vi "Do_ADAM_channel.vi"(4 "Scan Period":dbl format="%.2f", 5 "Previous Scan Value":dbl format="%.2f", 6 "Present scan array":dbl[](array[numeric]) format="%.2f", 7 "Value to Output":dbl format="%.2f", 8 "Ch Description":T1={"Ch Name"="", "Type"=enum."Test", "Function"=enum."Analogue Input", "Ch State"=enum."On", "Calibration type"=enum."Raw", "A"=0.0, "B"=0.0, "C"=0.0, "D"=0.0, "Comments"="", "Address"={"Main"=0, "Ch."=0, "Sub"=0, "Port Name"=""}, "String"="", "Duty"=0} {"Duty" format="%.0b"; "D" format="%#_5g"; "C" format="%#_5g"; "B" format="%#_5g"; "A" format="%#_5g"}, 9 "Ch names":string[](array[string])) -> (0 "Scan comment":string, 1 "Output":dbl format="%.3f")   [LabVIEW 2010]
uses:
  ADAM Client/Sub VIs/ADAM Controls/Ch_description_ADAM.ctl
  ADAM Client/Sub VIs/ADAM Controls/Module_type_ADAM.ctl
  ADAM Client/Sub VIs/ADAM Controls/Function_ADAM.ctl
  ADAM Client/Sub VIs/ADAM Controls/Channel_State.ctl
  ADAM Client/Sub VIs/ADAM Controls/Calib_type_ADAM.ctl
  ADAM Client/Sub VIs/ADAM Controls/Address.ctl
  ADAM Client/Sub VIs/ADAM Controls/Remember_value_mode.ctl
  ADAM Client/Sub VIs/ADAM Controls/Search_mode.ctl
  Anemometry/Anemometry Sub Vis/Controls/In_Range.ctl
  Anemometry/Anemometry Sub Vis/Globals/Gas_management_global.vi
  ADAM_Global.vi
  Anemometry/Anemometry Sub Vis/Globals/Constants_global.vi
panel:
  in  "Case Constant\n(See Context Help) 2":bool=TRUE
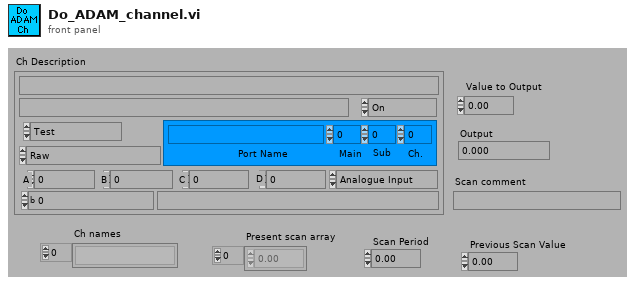
[diagram p1: front panel]
types:
  T1 = typedef "Ch_description_ADAM.ctl" = cluster{"Ch Name":string, "Type":T2, "Function":T3, "Ch State":T4, "Calibration type":T5, "A":dbl, "B":dbl, "C":dbl, "D":dbl, "Comments":string, "Address":T6, "String":string, "Duty":u16}
  T2 = typedef "Module_type_ADAM.ctl" = enum16{"4011", "4012", "4013", "4014", "4016", "4017", "4018", "4021", "4050", "4052", "4053", "4060", "4080", "5000", "5017", "5018", "5024", "5051", "5056", "5060", "6060", "Tracker", "WEST", "GILL", "JEM", "VICI", "Vaisala", "DRUCK", "Run VI Named:", "IR2100", "PPT", "Comparator", "VIRTUAL", "Hold Value", "Read A", "Read Ch", "Coded", "Client Info", "Web Client", "X10", "Test"}
  T3 = typedef "Function_ADAM.ctl" = enum16{"Analogue Input", "Digital Input", "Event counter", "Event rate", "Analogue Output", "Digital Output", "Relay Output"}
  T4 = typedef "Channel_State.ctl" = enum16{"On", "Off", "Always On", "Always Off"}
  T5 = typedef "Calib_type_ADAM.ctl" = enum16{"Raw", "Bx + A", "Cx^2 + Bx + A", "Dx^3 + Cx^2 + Bx + A", "In Band", "Hi-Tec Q", "Hi-Tec M_dot", "Text"}
  T6 = typedef "Address.ctl" = cluster{"Main":i32, "Ch.":i32, "Sub":i32, "Port Name":string}
  T7 = typedef "Remember_value_mode.ctl" = enum16{"Read only", "Read and Write"}
  T8 = typedef "Search_mode.ctl" = enum16{"Between times", "All Times"}
  T9 = typedef "In_Range.ctl" = enum16{"%", "±", "% & ±"}
  T10 = typedef "Valco_valve_ph.ctl" = u16
  T11 = cluster{"Centre Times":dbl[], "Output array":dbl[]}
  T12 = cluster{"Centre Times":dbl[], "Output array":dbl[]}[]
  T13 = typedef "LVDateTimeRec.ctl" = cluster{"fractional second":dbl, "second":i32, "minute":i32, "hour":i32, "day of month":i32, "month":i32, "year":i32, "day of week":i32, "day of year":i32, "DST":i32}
  T14 = typedef "Client_State_Cluster.ctl" = cluster{"Client Name":string, "Traverse level State":T15, "People to Email":string[], "Next Contact Time":dbl}
  T15 = typedef "Traverse_Level_State.ctl" = enum16{"Running", "Complete"}
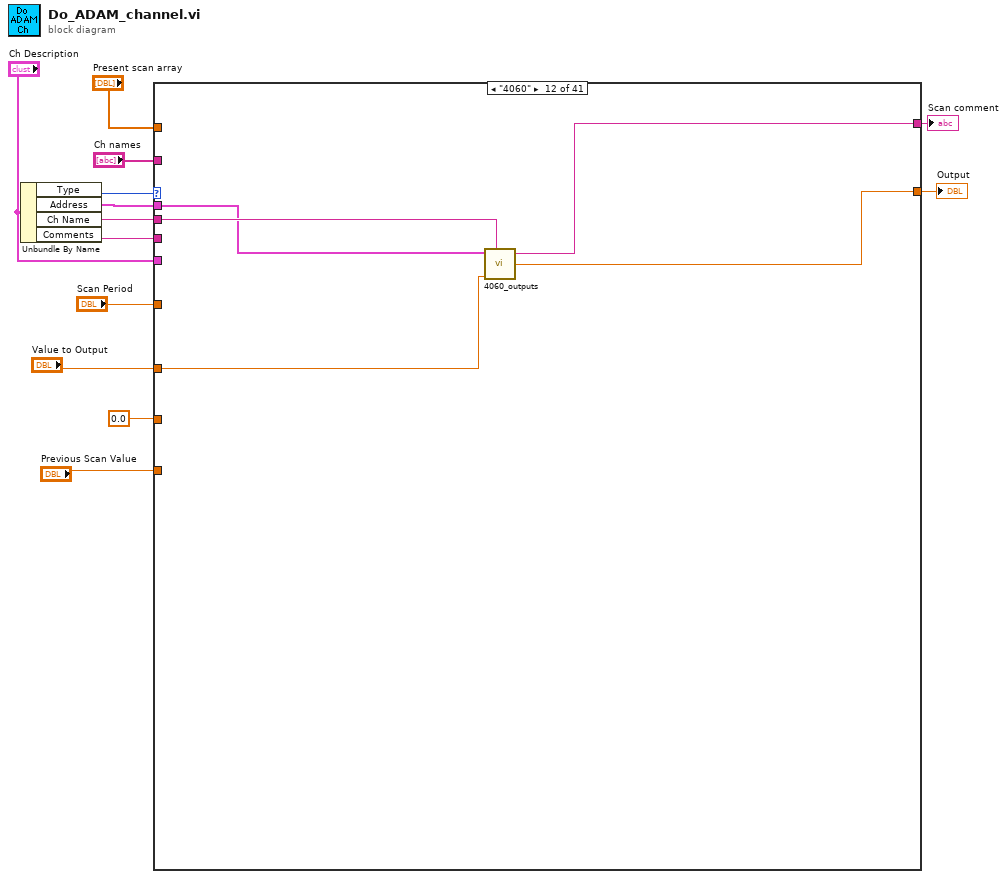
[diagram p0: block diagram]
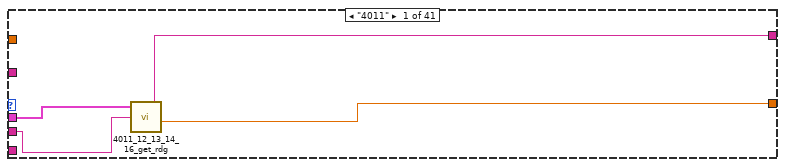
[diagram p2: hidden frame]
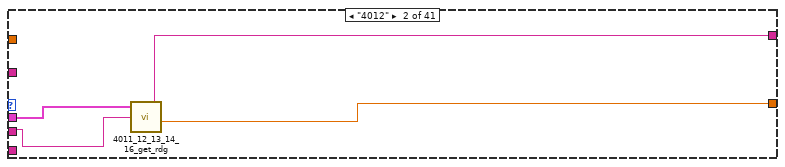
[diagram p3: hidden frame]
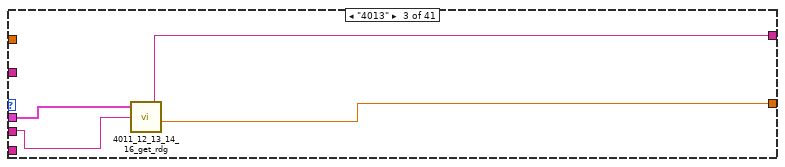
[diagram p4: hidden frame]
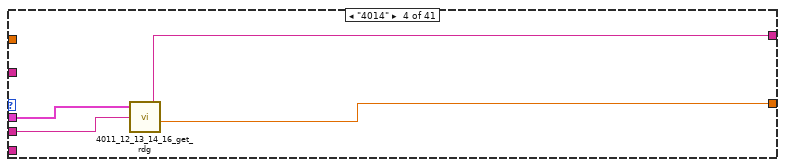
[diagram p5: hidden frame]
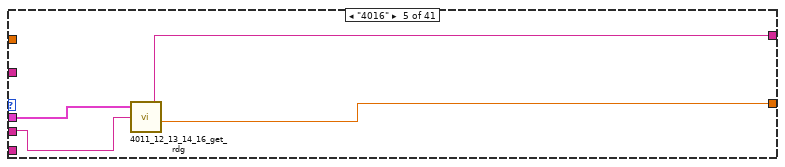
[diagram p6: hidden frame]
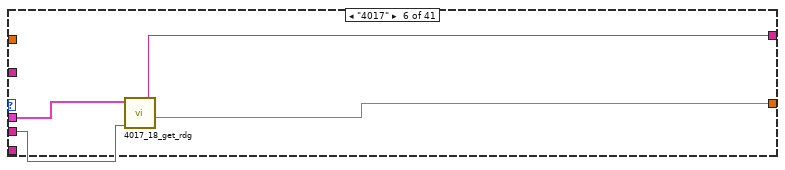
[diagram p7: hidden frame]
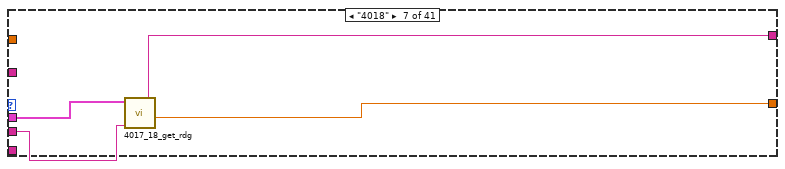
[diagram p8: hidden frame]
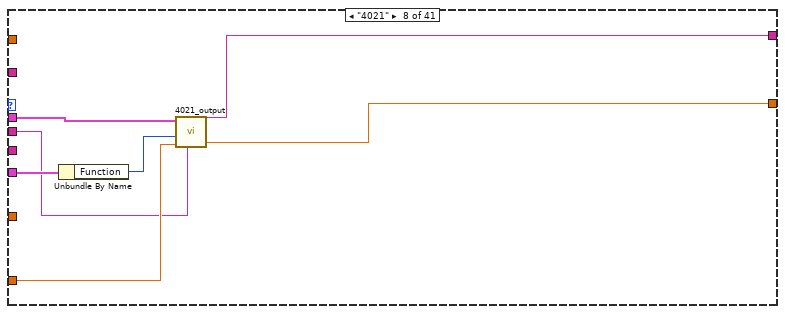
[diagram p9: hidden frame]
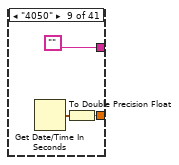
[diagram p10: hidden frame]
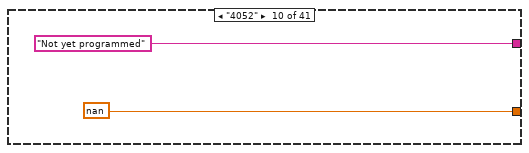
[diagram p11: hidden frame]
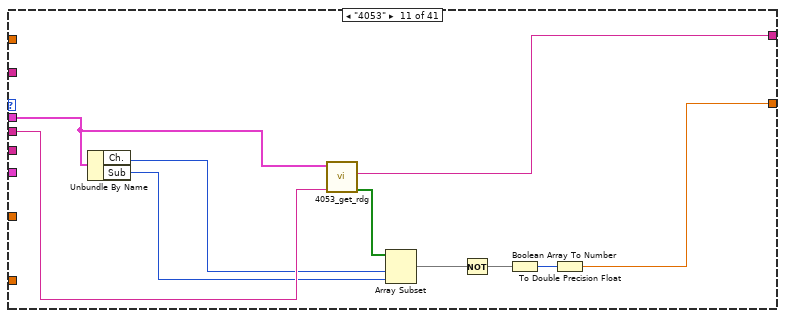
[diagram p12: hidden frame]
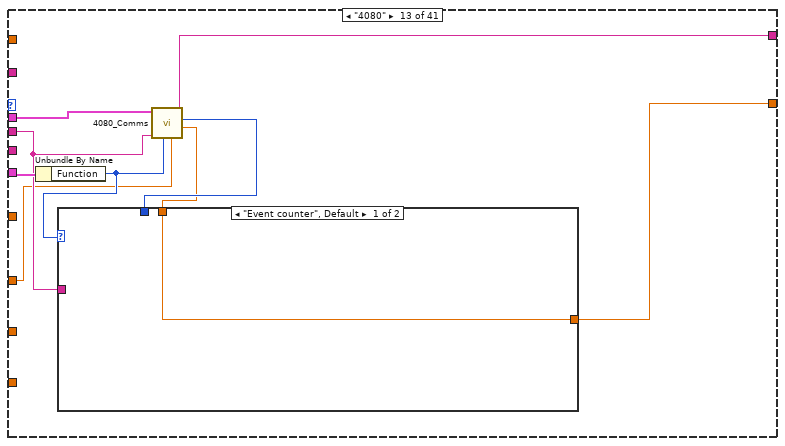
[diagram p13: hidden frame]
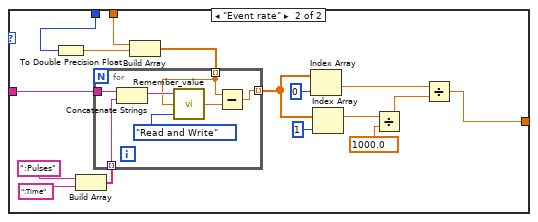
[diagram p14: hidden frame]
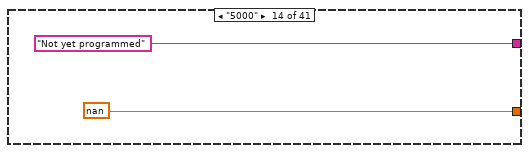
[diagram p15: hidden frame]
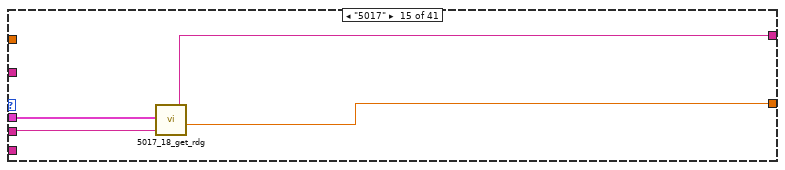
[diagram p16: hidden frame]
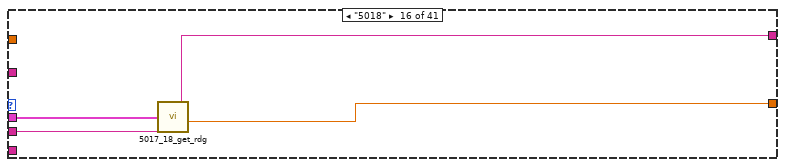
[diagram p17: hidden frame]
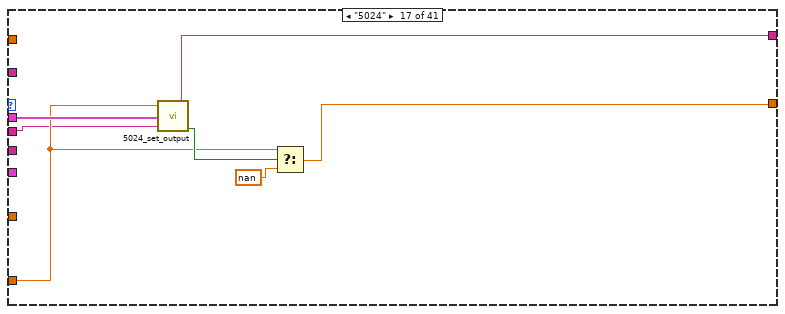
[diagram p18: hidden frame]
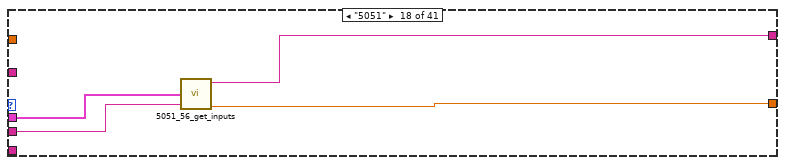
[diagram p19: hidden frame]
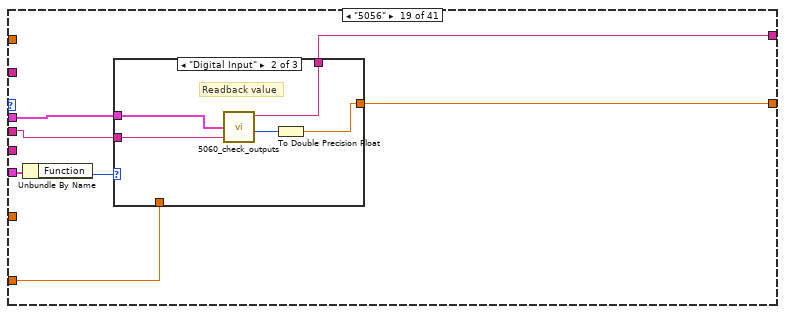
[diagram p20: hidden frame]
diagram:
  n1 = Unbundle By Name("Ch Description") -> ("Type"=w11:T2, "Address"=w10:T6, "Ch Name"=w2:string, "Comments"=w7:string)
  n2 = case shown="\"4060\"" w11 {
    tunnel: [w16 w20 w24 w28 w32 w36 w40 w47 w50 nan w57 w66 w75 nan w105 w109 w114 w120 w128 w149 w171 w190 nan w258 w271 w296 w335 nan w347 w378 w383 w384 w496 w920 w922 w926 w931 w943 w977 w1003 w1017] -> w8
    tunnel: [w17 w21 w25 w29 w33 w37 w41 w48 "" "Not yet programmed" w62 w67 w77 "Not yet programmed" w106 w110 w117 w121 w127 w150 w172 w192 "Not yet programmed" w257 w270 w288 w336 "Not yet programmed" w346 w379 w382 w405 w495 "" "" w927 "" "" w966 "" w1016] -> w5
    tunnel: w10 -> [w14 w18 w22 w26 w30 w34 w38 w42 _ _ w54 w65 w69 _ w107 w111 w118 w122 w126 w151 w173 w194 _ w255 w275 w293 w341 _ _ w377 w380 _ w487 _ _ _ _ _ _ w1012 w1015]
    tunnel: "Ch Description" -> [_ _ _ _ _ _ _ w46 _ _ _ _ w76 _ _ _ _ _ w125 w148 w170 w193 _ _ _ _ _ _ w352 _ _ w410 w489 _ w923 w928 _ _ _ _ _]
    tunnel: w2 -> [w15 w19 w23 w27 w31 w35 w39 w43 _ _ w63 w68 w72 _ w104 w108 w112 w119 w123 w145 w167 w191 _ w256 w273 w289 w340 _ _ _ w381 _ w492 _ _ _ _ w939 w973 _ w1014]
    tunnel: "Ch names" -> [_ _ _ _ _ _ _ _ _ _ _ _ _ _ _ _ _ _ _ _ _ _ _ _ _ _ _ _ w353 _ _ w409 w494 _ _ w929 _ _ _ _ _]
    tunnel: "Present scan array" -> [_ _ _ _ _ _ _ _ _ _ _ _ _ _ _ _ _ _ _ _ _ _ _ _ _ _ _ _ w350 _ _ w407 w493 _ _ w930 _ _ _ _ _]
    tunnel: w7 -> [_ _ _ _ _ _ _ _ _ _ _ _ _ _ _ _ _ _ _ _ _ _ _ _ _ _ _ _ w345 _ _ w411 _ _ _ _ _ _ _ _ _]
    tunnel: "Value to Output" -> [_ _ _ _ _ _ _ w44 _ _ _ w64 w70 _ _ _ w113 _ w124 w146 w168 w189 _ _ w259 w297 _ _ w351 _ _ _ _ _ _ _ _ _ _ w1007 _]
    tunnel: "Scan Period" -> [_ _ _ _ _ _ _ _ _ _ _ _ _ _ _ _ _ _ _ _ _ _ _ _ _ _ _ _ w348 _ _ _ w491 _ _ _ _ _ _ _ _]
    tunnel: "Previous Scan Value" -> [_ _ _ _ _ _ _ _ _ _ _ _ _ _ _ _ _ _ _ _ _ _ _ _ _ _ _ _ w349 _ _ w385 w490 w920 _ _ w931 _ _ _ _]
    tunnel: 0.0 -> [_ _ _ _ _ _ _ _ _ _ _ _ _ _ _ _ _ _ _ _ _ _ _ _ _ _ _ _ _ _ _ _ w488 _ _ _ _ _ _ _ _]
    frame "4011" {
      n3 = call "4011_12_13_14_16_get_rdg.vi"("Address"=w14, "Channel Name"=w15) -> ("Comment"=w17:string, "Reading"=w16:dbl)  [unwired: 1 in, 2 out]
    }
    frame "4012" {
      n4 = call "4011_12_13_14_16_get_rdg.vi"("Address"=w18, "Channel Name"=w19) -> ("Comment"=w21:string, "Reading"=w20:dbl)  [unwired: 1 in, 2 out]
    }
    frame "4013" {
      n5 = call "4011_12_13_14_16_get_rdg.vi"("Address"=w22, "Channel Name"=w23) -> ("Comment"=w25:string, "Reading"=w24:dbl)  [unwired: 1 in, 2 out]
    }
    frame "4014" {
      n6 = call "4011_12_13_14_16_get_rdg.vi"("Address"=w26, "Channel Name"=w27) -> ("Comment"=w29:string, "Reading"=w28:dbl)  [unwired: 1 in, 2 out]
    }
    frame "4016" {
      n7 = call "4011_12_13_14_16_get_rdg.vi"("Address"=w30, "Channel Name"=w31) -> ("Comment"=w33:string, "Reading"=w32:dbl)  [unwired: 1 in, 2 out]
    }
    frame "4017" {
      n8 = call "4017_18_get_rdg.vi"("Channel Name"=w35, "Address"=w34) -> ("Reading"=w36:dbl, "Comment"=w37:string)  [unwired: 2 in, 2 out]
    }
    frame "4018" {
      n9 = call "4017_18_get_rdg.vi"("Channel Name"=w39, "Address"=w38) -> ("Reading"=w40:dbl, "Comment"=w41:string)  [unwired: 2 in, 2 out]
    }
    frame "4021" {
      n10 = Unbundle By Name(w46) -> ("Function"=w45:T3)
      n11 = call "4021_output.vi"("Address"=w42, "Function"=w45, "Set to:"=w44, "Channel Name"=w43) -> ("Comment"=w48:string, "Reading"=w47:dbl)  [unwired: 1 in, 1 out]
    }
    frame "4050" {
      n12 = Get Date/Time In Seconds() -> (seconds since 1Jan1904=w49:timestamp)
      n13 = To Double Precision Float(number=w49) -> (double precision float=w50:dbl)
    }
    frame "4052" {
    }
    frame "4053" {
      n14 = Unbundle By Name(w54) -> ("Ch."=w55:i32, "Sub"=w61:i32)
      n15 = call "4053_get_rdg.vi"("Channel Name"=w63, "Address"=w54) -> ("Boolean array"=w60:bool[], "Comment"=w62:string)  [unwired: 2 in, 2 out]
      n16 = Array Subset(array=w60, index=w55, length=w61) -> (w59:bool[])
      n17 = Not(x=w59) -> (.not. x?=w56:bool[])
      n18 = Boolean Array To Number(Boolean array=w56) -> (number=w58:u32)
      n19 = To Double Precision Float(number=w58) -> (double precision float=w57:dbl)
    }
    frame "4060" {
      n20 = call "4060_outputs.vi"("Address"=w65, "Value to Output"=w64, "Channel Name"=w68) -> ("Comment"=w67:string, "Reading"=w66:dbl)  [unwired: 2 in, 1 out]
    }
    frame "4080" {
      n21 = Unbundle By Name(w76) -> ("Function"=w71:T3)
      n22 = call "4080_Comms.vi"("Value to display"=w70, "Function"=w71, "Channel Name"=w72, "Address"=w69) -> ("Reading"=w73:dbl, "millisecond timer value"=w74:u32, "Comment"=w77:string)  [unwired: 2 in, 1 out]
      n23 = case shown="\"Event counter\", Default" w71 {
        tunnel: w72 -> [_ w94]
        tunnel: w74 -> [_ w87]
        tunnel: [w78 w79] -> w75
        tunnel: w73 -> [w78 w88]
        frame "Event counter", Default {
        }
        frame "Event rate" {
          n24 = To Double Precision Float(number=w87) -> (double precision float=w86:dbl)
          n25 = Build Array(":Pulses", ":Time") -> (w89:string[])
          n26 = Build Array(w88, w86) -> (w85:dbl[])
          n27 = for {
            tunnel: w94 -> [w98]
            tunnel: [w99] -> w82 mode=indexing
            tunnel: w89 -> [w96] mode=indexing
            tunnel: w85 -> [w95] mode=indexing
            n28 = Concatenate Strings(w98, w96) -> (w97:string)
            n29 = call "Remember_value.vi"("Mode"=Remember_value_mode."Read and Write", "Input Value"=w95, "Ch name"=w97) -> ("Output Value"=w100:dbl)
            n30 = Subtract(x=w95, y=w100) -> (x-y=w99:dbl)
          }
          n31 = Index Array(array=w82, index=0) -> (element=w80:dbl)
          n32 = Index Array(array=w82, index=1) -> (element=w81:dbl)
          n33 = Divide(x=w81, y=1000.0) -> (x/y=w92:dbl)
          n34 = Divide(x=w80, y=w92) -> (x/y=w79:dbl)
        }
      }
    }
    frame "5000" {
    }
    frame "5017" {
      n35 = call "5017_18_get_rdg.vi"("Address (all reqd.)"=w107, "Channel Name"=w104) -> ("Comment"=w106:string, "Reading"=w105:dbl)  [unwired: 3 out]
    }
    frame "5018" {
      n36 = call "5017_18_get_rdg.vi"("Address (all reqd.)"=w111, "Channel Name"=w108) -> ("Comment"=w110:string, "Reading"=w109:dbl)  [unwired: 3 out]
    }
    frame "5024" {
      n37 = call "5024_set_output.vi"("Set to:"=w113, "Address (all reqd.)"=w118, "Channel Name"=w112) -> ("Comment"=w117:string, "Good Reply"=w115:bool)  [unwired: 2 out]
      n38 = Select(t=w113, s=w115, f=nan) -> (s? t:f=w114:dbl)
    }
    frame "5051" {
      n39 = call "5051_56_get_inputs.vi"("Address (Main, Sub reqd.)"=w122, "Channel Name"=w119) -> ("Comment"=w121:string, "Single output"=w120:dbl)  [unwired: 3 out]
    }
    frame "5056" {
      n40 = Unbundle By Name(w125) -> ("Function"=w129:T3)
      n41 = case shown="\"Digital Input\"" w129 {
        tunnel: w126 -> [_ w135 w144]
        tunnel: ["This function is not available" w136 w142] -> w127
        tunnel: [nan ("A") w133 w139] -> w128
        tunnel: w124 -> [_ _ w138]
        tunnel: w123 -> [_ w132 w137]
        frame "Analogue Input", Default {
        }
        frame "Digital Input" {
          # "Readback value"
          n42 = call "5060_check_outputs.vi"("Address (Main, Sub reqd.)"=w135, "Channel Name"=w132) -> ("Comment"=w136:string, "Single Channel"=w134:i16)  [unwired: 3 out]
          n43 = To Double Precision Float(number=w134) -> (double precision float=w133:dbl)
        }
        frame "Relay Output" {
          # "Sets single o/p channel"
          n44 = Greater Than 0?(x=w138) -> (x > 0?=w143:bool)
          n45 = call "5056_60_set_single_output.vi"("Channel Name"=w137, "Address (all reqd.)"=w144, "Set state:"=w143) -> ("Comment"=w142:string, "Good Reply"=w141:bool)  [unwired: 2 out]
          n46 = Select(t=w138, s=w141, f=nan) -> (s? t:f=w139:dbl)
        }
      }
    }
    frame "5060" {
      n47 = Unbundle By Name(w148) -> ("Function"=w147:T3)
      n48 = case shown="\"Relay Output\"" w147 {
        tunnel: w151 -> [_ w157 w166]
        tunnel: ["This function is not available" w158 w164] -> w150
        tunnel: [nan ("A") w155 w161] -> w149
        tunnel: w146 -> [_ _ w160]
        tunnel: w145 -> [_ w154 w159]
        frame "Analogue Input", Default {
        }
        frame "Digital Input" {
          # "Readback value"
          n49 = call "5060_check_outputs.vi"("Address (Main, Sub reqd.)"=w157, "Channel Name"=w154) -> ("Comment"=w158:string, "Single Channel"=w156:i16)  [unwired: 3 out]
          n50 = To Double Precision Float(number=w156) -> (double precision float=w155:dbl)
        }
        frame "Relay Output" {
          # "Sets single o/p channel"
          n51 = Greater Than 0?(x=w160) -> (x > 0?=w165:bool)
          n52 = call "5056_60_set_single_output.vi"("Channel Name"=w159, "Address (all reqd.)"=w166, "Set state:"=w165) -> ("Comment"=w164:string, "Good Reply"=w163:bool)  [unwired: 2 out]
          n53 = Select(t=w160, s=w163, f=nan) -> (s? t:f=w161:dbl)
        }
      }
    }
    frame "6060" {
      n54 = Unbundle By Name(w170) -> ("Function"=w169:T3)
      n55 = case shown="\"Digital Input\"" w169 {
        tunnel: w173 -> [_ w179 w188]
        tunnel: ["This function is not available" w180 w186] -> w172
        tunnel: [nan ("A") w177 w183] -> w171
        tunnel: w168 -> [_ _ w182]
        tunnel: w167 -> [_ w176 w181]
        frame "Analogue Input", Default {
        }
        frame "Digital Input" {
          n56 = call "6060_read_all_I-O.vi"("Address (Main, Sub reqd.)"=w179, "Channel Name"=w176) -> ("Comment"=w180:string, "Single Input Channel"=w178:i16)  [unwired: 3 out]
          n57 = To Double Precision Float(number=w178) -> (double precision float=w177:dbl)
        }
        frame "Relay Output" {
          # "Sets single o/p channel"
          n58 = Greater Than 0?(x=w182) -> (x > 0?=w187:bool)
          n59 = call "6060_set_single_output.vi"("Channel Name"=w181, "Address (Main, Ch requd.)"=w188, "Set state:"=w187) -> ("Comment"=w186:string, "Good Reply"=w185:bool)  [unwired: 2 out]
          n60 = Select(t=w182, s=w185, f=nan) -> (s? t:f=w183:dbl)
        }
      }
    }
    frame "Tracker" {
      n61 = while {
        tunnel: w194 -> [w218]
        tunnel: w193 -> [w217]
        tunnel: [w211] -> w192
        tunnel: w191 -> [w210]
        tunnel: [w204] -> w190
        tunnel: w189 -> [w203]
        i -> [w200]
        stop <- w197 continue-if-true
        n62 = Unbundle By Name(w217) -> ("Function"=w216:T3)
        n63 = Unbundle By Name(w218) -> ("Port Name"=w215:string, "Ch."=w206:i32, "Main"=w214:i32, "Sub"=w213:i32)
        n64 = case shown="\"Analogue Output\"" w216 {
          tunnel: [enum16{"Set", "Read"}."Set" ("Set") enum16{"Set", "Read"}."Set" ("Set") enum16{"Set", "Read"}."Set" ("Set") enum16{"Set", "Read"}."Set" ("Set") enum16{"Set", "Read"}."Set" ("Set") enum16{"Set", "Read"}."Read" ("Set") enum16{"Set", "Read"}."Read" ("Set")] -> w201
          tunnel: [enum16{"Logic", "Analogue"}."Analogue" ("Analogue") enum16{"Logic", "Analogue"}."Logic" ("Analogue") enum16{"Logic", "Analogue"}."Logic" ("Analogue") enum16{"Logic", "Analogue"}."Logic" ("Analogue") enum16{"Logic", "Analogue"}."Logic" ("Analogue") enum16{"Logic", "Analogue"}."Logic" ("Analogue") enum16{"Logic", "Analogue"}."Analogue" ("Analogue")] -> w212
          frame "Analogue Output" {
          }
          frame "Digital Output" {
          }
          frame "Relay Output" {
          }
          frame "Event rate" {
          }
          frame "Event counter" {
          }
          frame "Digital Input" {
          }
          frame "Analogue Input" {
          }
        }
        n65 = call "TalkTracker.vi"("PORT NAME"=w215, "Set"=w201, "Channel Name"=w210, "Value to set"=w203, "MODULE ADDRESS"=w214, "LOCATION"=w206, "NO. LOCATIONS"=w213, "Analogue"=w212) -> ("Response"=w208:string, "Good Set?"=w195:bool, "Comment out"=w211:string)  [unwired: 1 in, 4 out]
        n66 = Match Pattern(string=w208, regular expression="\r\n") -> (before substring=w207:string)  [unwired: 4 out]
        n67 = case shown="\"Set\"" w201 {
          tunnel: w207 -> [_ w230]
          tunnel: [w222 w229] -> w205
          tunnel: w203 -> [w224 _]
          tunnel: nan ("Reading") -> [w223 w228]
          tunnel: [w221 w226] -> w198
          tunnel: [0 ("y") 1 ("y")] -> w196
          tunnel: w195 -> [w219 _]
          frame "Set" {
            n68 = Not(x=w219) -> (.not. x?=w221:bool)
            n69 = Select(t=w224, s=w219, f=w223) -> (s? t:f=w222:dbl)
          }
          frame "Read" {
            n70 = String Length(string=w230) -> (length=w232:i32)
            n71 = Fract/Exp String To Number(string=w230, default (0 dbl)=w228) -> (offset past number=w233:i32, number=w231:dbl)  [unwired: 2 out]
            n72 = Equal?(x=w232, y=w233) -> (x = y?=w227:bool)
            n73 = Not(x=w227) -> (.not. x?=w226:bool)
            n74 = Select(t=w231, s=w227, f=w228) -> (s? t:f=w229:dbl)
          }
        }
        n75 = case shown="0, Default" w206 {
          tunnel: w205 -> [w234 w237]
          tunnel: [w234 w235] -> w204
          frame 0, Default {
          }
          frame 283 {
            n76 = Equal To 0?(x=w237) -> (x = 0?=w238:bool)
            n77 = Select(t=nan ("Reading"), s=w238, f=w237) -> (s? t:f=w235:dbl)
          }
        }
        n78 = Less?(x=w200, y=w196) -> (x < y?=w199:bool)
        n79 = And(x=w198, y=w199) -> (x .and. y?=w197:bool)
      }
    }
    frame "WEST" {
    }
    frame "GILL" {
      n80 = call "Gill_get_rdg.vi"("Channel Name"=w256, "Address"=w255) -> ("Output"=w258:dbl, "Status note"=w257:string)  [unwired: 2 in, 2 out]
    }
    frame "JEM" {
      n81 = Unbundle By Name(w275) -> ("Main"=w262:i32, "Ch."=w261:i32, "Port Name"=w274:string)
      n82 = case shown="0, Default" w261 {
        tunnel: [i16[] [-3, -2, -1, 0, 14, 29, 43, 57, 71, 86, 100] i16[] [0, 20, 40, 60, 80, 100, 120]] -> w265
        tunnel: [u8[] [10, 50, 80, 100, 120, 140, 160, 180, 200, 220, 240] u8[] [20, 50, 90, 130, 160, 200, 230]] -> w266
        frame 0, Default {
        }
        frame 1 {
        }
      }
      n83 = Add(x=w262, y=w261) -> (x+y=w260:i32)
      n84 = Threshold 1D Array(2:w259, 3:w265) -> (0:w268:dbl)  [unwired: 1 out]
      n85 = Round To Nearest(number=w268) -> (nearest integer value=w269:dbl)
      n86 = To Long Integer(number=w269) -> (32bit integer=w267:i32)
      n87 = Index Array(array=w266, index=w267) -> (element=w264:u8)
      n88 = call "DMX.vi"("Port Name"=w274, "DMX channel no."=w260, "Set value:"=w264, "Channel Name"=w273) -> ("error"=w272:bool)  [unwired: 2 out]
      n89 = Index Array(array=w265, index=w267) -> (element=w263:i16)
      n90 = case shown="False" w272 {
        tunnel: [w276 nan] -> w271
        tunnel: ["" "Comms Error"] -> w270
        tunnel: w263 -> [w278 _]
        frame False {
          n91 = To Double Precision Float(number=w278) -> (double precision float=w276:dbl)
        }
        frame True {
        }
      }
    }
    frame "VICI" {
      n92 = To Long Integer(number=w297) -> (32bit integer=w292:i32)
      n93 = Unbundle By Name(w293) -> ("Port Name"=w295:string, "Ch."=w294:i32)
      n94 = call "Valco_Valve_Position.vi"("Channel Name"=w289, "Valve Number"=w294, "Port Name"=w295, "Requested Posn."=w292) -> ("Error Message"=w287:string, "Achieved Posn."=w290:T10)  [unwired: 2 out]
      n95 = Empty String/Path?(string/path=w287) -> ()  [unwired: 1 out]
      n96 = case shown="True" TRUE {
        tunnel: w293 -> [w304 _]
        tunnel: w292 -> [w303 _]
        tunnel: [w302 w334] -> w291
        tunnel: w290 -> [_ w334]
        tunnel: w289 -> [w301 _]
        tunnel: [w300 w333] -> w288
        tunnel: w287 -> [_ w333]
        tunnel: w287 -> [w299 _]
        tunnel: "X10" ("Port Name") -> [w298 _]
        frame False {
          n97 = stacked-sequence {
            tunnel: w304 -> [_ _ _ _ _ w325]
            tunnel: w303 -> [_ _ _ _ _ w321]
            tunnel: [_ _ _ _ _ w324] -> w302
            tunnel: w301 -> [_ _ _ _ _ w323]
            tunnel: [_ _ _ _ _ w322] -> w300
            tunnel: w299 -> [_ w310 _ _ _ _]
            tunnel: w298 -> [w305 _ _ w313 _ _]
            frame #0 {
              w307 = 3 items=["-----", "A", "B", "C", "D", "E", "F", "G", "H", "I", "J", "K", "L", "M", "N", "O", "P"] ("House Code")
              n98 = call "X10control.vi"("Port Name"=w305, "Power Request (ON)"=FALSE, "House Code"=w307, "Unit No."=5) -> ()  [unwired: 6 out]
            }
            frame #1 {
              n99 = call "Server_Emails.vi"("Message"=w310, "Contact All clients?"=TRUE, "Subject"="Powering Down FID Valve" ("Error Type")) -> ()  [unwired: 2 in, 3 out]
            }
            frame #2 {
              n100 = Wait (ms)(milliseconds to wait=u32 20000) -> ()  [unwired: 1 out]
            }
            frame #3 {
              w315 = 3 items=["-----", "A", "B", "C", "D", "E", "F", "G", "H", "I", "J", "K", "L", "M", "N", "O", "P"] ("House Code")
              n101 = call "X10control.vi"("Port Name"=w313, "Power Request (ON)"=TRUE, "House Code"=w315, "Unit No."=5) -> ()  [unwired: 6 out]
            }
            frame #4 {
              n102 = Wait (ms)(milliseconds to wait=u32 5000) -> ()  [unwired: 1 out]
            }
            frame #5 {
              n103 = Build Array(1 ("element"), 2 ("element"), w321) -> (w318:i32[])
              n104 = for {
                tunnel: w325 -> [w330]
                tunnel: [w329] -> w324
                tunnel: w323 -> [w328]
                tunnel: [w327] -> w322
                tunnel: w318 -> [w326] mode=indexing
                n105 = Unbundle By Name(w330) -> ("Port Name"=w331:string, "Ch."=w332:i32)
                n106 = call "Valco_Valve_Position.vi"("Channel Name"=w328, "Valve Number"=w332, "Port Name"=w331, "Requested Posn."=w326) -> ("Error Message"=w327:string, "Achieved Posn."=w329:T10)  [unwired: 2 out]
              }
            }
          }
        }
        frame True {
        }
      }
      n107 = To Double Precision Float(number=w291) -> (double precision float=w296:dbl)
    }
    frame "Vaisala" {
      n108 = Unbundle By Name(w341) -> ("Main"=w337:i32, "Ch."=w338:i32, "Port Name"=w339:string)
      n109 = call "HMP231.vi"("Channel Name"=w340, "Port Name"=w339, "Channel"=w338, "Address"=w337) -> ("Output"=w335:dbl, "Status note"=w336:string)  [unwired: 2 out]
    }
    frame "DRUCK" {
    }
    frame "Run VI Named:" {
      n110 = Current VI's Path() -> (path=w362:path)
      n111 = Strip Path(path=w362) -> (stripped path=w363:path)  [unwired: 1 out]
      n112 = call <vilib>:"Trim Whitespace.vi"("string"=w345) -> ("trimmed string"=w344:string)  [unwired: 1 in]
      n113 = Strip Path(path=w363) -> (stripped path=w364:path)  [unwired: 1 out]
      n114 = Build Path(base path=w364, name or relative path="Run_vi_named") -> (appended path=w366:path)
      n115 = Build Path(base path=w366, name or relative path=w344) -> (appended path=w361:path)
      n116 = Open VI Reference(type specifier VI Refnum (for type only)=refnum<vi> refnum, vi path=w361) -> (vi reference=w357:refnum<vi>, error out=w356:errorcluster)  [unwired: 1 in, 3 out]
      n117 = property class="VI Interface Type 3"(reference=w357, error in=w356) -> (reference out=w359:refnum<vi>, error out=w358:errorcluster, "Front Panel Window:Open"=w360:bool)
      n118 = case shown="False" w360 {
        tunnel: w359 -> [w374 w376]
        tunnel: w358 -> [w373 w375]
        tunnel: [w372 w376] -> w355
        tunnel: [w370 w375] -> w354
        frame False {
          n119 = property class="VI Interface Type 3"(reference=w374, error in=w373, "Front Panel Window:Open"=TRUE) -> (reference out=w372:refnum<vi>, error out=w370:errorcluster)
        }
        frame True {
        }
      }
      n120 = call-by-ref "?"(reference=w355, error in=w354, "Scan Period"=w348, "Previous Scan Value"=w349, "Present scan array"=w350, "Value to Output"=w351, "Ch Description"=w352, "Ch names"=w353) -> (reference out=w368:refnum<vi>, error out=w369:errorcluster, "Scan comment"=w346:string, "Output"=w347:dbl)  [unwired: 2 in]
      n121 = Close Reference(reference=w368, error in (no error)=w369) -> ()  [unwired: 1 out]
    }
    frame "IR2100" {
      n122 = call "IR2100_get_rdg.vi"("Address"=w377) -> ("Comment"=w379:string, "Reading"=w378:dbl)  [unwired: 2 in, 2 out]
    }
    frame "PPT" {
      n123 = call "PPT_get_rdg.vi"("Channel Name"=w381, "Address"=w380) -> ("Reading"=w383:dbl, "Comment"=w382:string)  [unwired: 2 in, 2 out]
    }
    frame "Comparator" {
      # "A Warn if above this value\nB Warn if below this value\nC  Hysteresis margin\nD is the averaging time in minutes\nComments   is Channel name to check"
      n124 = Unbundle By Name(w410) -> ("D"=w393:dbl)
      n125 = Match Pattern(string=w411, regular expression=":::" ("String to match")) -> (before substring=w408:string)  [unwired: 4 out]
      n126 = call "Read_value_of_earlier_Ch.vi"("Desired Ch to Read"=w408, "Ch names"=w409, "Present scan array"=w407) -> ("Value"=w392:dbl, "Scan comment"=w406:string)  [unwired: 1 in]
      n127 = Equal?(x=w385, y=1.0) -> (x = y?=w401:bool)
      n128 = Unbundle By Name(w410) -> ("A"=w404:dbl, "B"=w403:dbl, "C"=w402:dbl)
      n129 = Equal To 0?(x=w393) -> (x = 0?=w391:bool)
      n130 = case shown="True" w401 {
        tunnel: [w417 w422] -> w399
        tunnel: w404 -> [w417 w421]
        tunnel: w403 -> [w416 w420]
        tunnel: [w416 w418] -> w400
        tunnel: w402 -> [_ w419]
        frame False {
        }
        frame True {
          n131 = Subtract(x=w421, y=w419) -> (x-y=w422:dbl)
          n132 = Add(x=w420, y=w419) -> (x+y=w418:dbl)
        }
      }
      n133 = case shown="False" w391 {
        tunnel: [w427 w430] -> w414
        tunnel: w408 -> [w429 _]
        tunnel: [w425 w431] -> w390
        tunnel: w393 -> [w423 _]
        tunnel: w392 -> [_ w431]
        tunnel: w406 -> [w427 w430]
        frame False {
          n134 = Build Array(w429) -> (w424:string[])
          n135 = call "Get_Channel_averages.vi"("Desired Ch Names"=w424, "Averaging time (mins)"=w423) -> ("number"=w426:dbl[])  [unwired: 1 in, 2 out]
          n136 = Index Array(array=w426, index=0) -> (element=w425:dbl)
        }
        frame True {
        }
      }
      n137 = Not(x=w401) -> (.not. x?=w394:bool)
      n138 = In Range and Coerce(upper limit=w399, x=w390, lower limit=w400) -> (In Range?=w395:bool)  [unwired: 1 out]
      n139 = Greater?(x=w390, y=w399) -> (0:w398:bool)
      n140 = Not A Number/Path/Refnum?(number/path/refnum=w390) -> (NaN/Path/Refnum?=w387:bool)
      n141 = Equal?(x=w395, y=w394) -> (x = y?=w389:bool)
      n142 = Or(x=w389, y=w387) -> (x .or. y?=w388:bool)
      n143 = case shown="False" w388 {
        tunnel: w408 -> [w438 _]
        tunnel: w399 -> [w437 _]
        tunnel: w410 -> [w436 _]
        tunnel: w400 -> [w435 _]
        tunnel: w395 -> [w434 _]
        tunnel: w390 -> [w433 _]
        tunnel: w398 -> [w432 _]
        frame False {
          n144 = stacked-sequence {
            seq-local: [w444 _ _ _ _] -> [_ _ _ w485 _]
            seq-local: [_ w464 _ _ _] -> [_ _ _ w482 _]
            seq-local: [w442 _ _ _ _] -> [_ _ _ w478 _]
            tunnel: w438 -> [w446 w472 _ w484 _]
            tunnel: w437 -> [w445 _ _ _ _]
            tunnel: w436 -> [_ _ w477 w486 _]
            tunnel: w435 -> [w443 _ _ _ _]
            tunnel: w434 -> [w441 _ _ _ _]
            tunnel: w433 -> [w440 _ _ _ _]
            tunnel: w432 -> [w439 _ _ _ _]
            frame #0 {
              n145 = case shown="False" w441 {
                tunnel: w446 -> [w451 w462]
                tunnel: w445 -> [_ w455]
                tunnel: [w449 w461] -> w444
                tunnel: w443 -> [_ w454]
                tunnel: ["OK " ""] -> w442
                tunnel: w440 -> [w447 _]
                tunnel: w439 -> [_ w452]
                frame True {
                  n146 = Format Into String(format string="The channel named %s is now  %.3f" ("Format String"), w451, w447) -> (resulting string=w449:string)  [unwired: 2 in, 1 out]
                }
                frame False {
                  n147 = Select(t=w455, s=w452, f=w454) -> (s? t:f=w453:dbl)
                  n148 = Select(t="greater", s=w452, f="less") -> (s? t:f=w457:string)
                  n149 = Format Into String(format string="%s is %s than %.3f" ("Format String"), w462, w457, w453) -> (resulting string=w461:string)  [unwired: 2 in, 1 out]
                }
              }
            }
            frame #1 {
              n150 = Build Array(w472) -> (w471:string[])
              n151 = call "Channel_Names_and_indicies.vi"("All Active Channels"=FALSE, "Desired Ch Names"=w471) -> ("Indicies"=w469:i32[])  [unwired: 1 out]
              n152 = call "Specified_Channels_server.vi"("Mode"=Search_mode."All Times", "Requested channels"=w469) -> ("Output array"=w467:dbl[][], "Centre Times"=w463:dbl[])  [unwired: 3 in, 3 out]
              n153 = Index Array(array=w467, index (row)=0) -> (element=w465:dbl[])  [unwired: 1 in]
              n154 = Bundle("Centre Times"=w463, "Output array"=w465) -> (w468:T11)  [unwired: 1 out]
              n155 = Build Array(w468) -> (w464:T12)
            }
            frame #2 {
              w475 = TRUE  # Contact All clients?
              n156 = Unbundle By Name(w477) -> ("String"=w476:string)
              n157 = call "Get_array_values_fr_String.vi"("String Value"=w476) -> ("String array"=w474:string[])  [unwired: 1 out]
              n158 = call "Client_email_addresses.vi"("Extra People to Email"=w474, "Contact All clients?"=w475) -> ()  [unwired: 1 in]
            }
            frame #3 {
              n159 = Unbundle By Name(w486) -> ("Ch Name"=w479:string)
              n160 = Build Array(w484) -> (w483:string[])
              n161 = Concatenate Strings(w478, w479) -> (w480:string)
              n162 = call "Email_Attachment_Plot.vi"("X axis name"="Time", "XY Graph"=w482, "Series Names"=w483, "message"=w485, "subject ([No Subject])"=w480) -> ()  [unwired: 1 in, 1 out]
            }
            frame #4 {
            }
          }
        }
        frame True {
        }
      }
      n163 = Concatenate Strings(w414, "") -> (w405:string)
      n164 = Select(t=0.0, s=w395, f=1.0) -> (s? t:f=w386:dbl)
      n165 = Select(t=w385, s=w387, f=w386) -> (s? t:f=w384:dbl)
    }
    frame "VIRTUAL" {
      n166 = case shown="\"Laser:Cooling_Water:Delta_T\"" w492 {
        tunnel: [w506 w520 w534 w556 w571 w582 w598 w629 w656 w691 w700 w717 w770 w796 w823 w843] -> w496
        tunnel: [w497 w526 w532 w560 w565 w580 w607 "" w660 w685 w694 w714 w769 w795 "" w844] -> w495
        tunnel: w494 -> [w503 w528 w538 w562 w567 w585 w609 w633 w662 w687 w696 w715 w775 w800 _ w846]
        tunnel: w493 -> [w504 w527 w539 w561 w566 w586 w608 w634 w663 w686 w695 w716 w777 w802 _ w845]
        tunnel: w492 -> [w501 _ _ _ _ _ _ _ _ _ _ w703 _ _ w818 _]
        tunnel: w491 -> [w502 _ _ _ _ _ _ _ _ _ _ _ w767 w794 w823 w842]
        tunnel: w490 -> [w505 _ _ _ _ _ _ _ _ _ _ w718 w771 w797 _ w841]
        tunnel: w489 -> [_ _ w530 _ _ _ _ _ _ _ _ w709 _ _ _ _]
        tunnel: w488 -> [_ w519 _ _ _ w579 _ _ _ _ _ _ _ _ _ _]
        tunnel: w487 -> [_ _ _ _ _ _ _ _ _ _ _ _ _ _ _ _]
        frame "GMU:Remaining:", Default {
          n167 = Match Pattern(string=w501, regular expression="GMU:Remaining:" ("String to match")) -> (match substring=w499:string)  [unwired: 4 out]
          n168 = Empty String/Path?(string/path=w499) -> (empty?=w498:bool)
          n169 = case shown="False" w498 {
            tunnel: [w513 nan] -> w506
            tunnel: w505 -> [w512 _]
            tunnel: w504 -> [w511 _]
            tunnel: w503 -> [w510 _]
            tunnel: w502 -> [w509 _]
            tunnel: w501 -> [w508 _]
            tunnel: [w507 w515] -> w497
            frame False {
              n170 = call "Update_Rem_gas.vi"("Scan Period (s)"=w509, "Gas Remaining in"=w512, "Ch name"=w508, "Ch names"=w510, "Present scan array"=w511) -> ("Gas Remaining out"=w513:dbl, "Comments"=w507:string)  [unwired: 1 out]
            }
            frame True {
              n171 = Current VI's Path() -> (path=w517:path)
              n172 = Path To String(path=w517) -> (string=w516:string)
              n173 = Concatenate Strings(" was not matched in ", w516) -> (w515:string)
            }
          }
        }
        frame "GMU:Source:Meas Q" {
          n174 = call "Calculate_Release_Flowrates.vi"("Ch names"=w528, "Units"=enum16{"Q l/min", "M_dot Kg/min"}."Q l/min", "Present scan array"=w527) -> ("Trace"=w524:dbl, "Carrier"=w525:dbl, "Scan comments"=w526:string)
          n175 = Add(x=w525, y=w524) -> (x+y=w521:dbl)
          n176 = Not Equal To 0?(x=w521) -> (x != 0?=w522:bool)
          n177 = Select(t=w521, s=w522, f=w519) -> (s? t:f=w520:dbl)
        }
        frame "GMU:Detector:Strength" {
          n178 = Unbundle By Name(w530) -> ("C"=w529:dbl)
          n179 = call "Read_value_of_earlier_Ch.vi"("Desired Ch to Read"="GMU:Detector:Meas Current", "Ch names"=w538, "Present scan array"=w539) -> ("Value"=w535:dbl, "Scan comment"=w533:string)  [unwired: 1 in]
          n180 = Greater?(x=w535, y=w529) -> (0:w536:bool)
          n181 = case shown="True" w536 {
            tunnel: w530 -> [_ w551]
            tunnel: w535 -> [_ w546]
            tunnel: [100.0 ("Eng Values") w544] -> w534
            tunnel: ["Fault" w547] -> w531
            frame False {
            }
            frame True {
              n182 = Unbundle By Name(w551) -> ("D"=w542:dbl, "A"=w550:dbl, "B"=w549:dbl)
              n183 = Less?(x=w546, y=w542) -> (x < y?=w545:bool)
              n184 = Build Array(w550, w549) -> (w548:dbl[])
              n185 = call "Polynomial_convert.vi"("Calib constants"=w548, "Voltage"=w546) -> ("Eng Values"=w543:dbl)  [unwired: 4 out]
              n186 = case shown="True" w545 {
                tunnel: ["Saturated" ""] -> w547
                tunnel: [100.0 ("Eng Values") w554] -> w544
                tunnel: w543 -> [_ w554]
                frame False {
                }
                frame True {
                }
              }
            }
          }
          n187 = Concatenate Strings(w533, w531) -> (w532:string)
        }
        frame "GMU:Source:Meas M_dot" {
          n188 = call "Calculate_Release_Flowrates.vi"("Ch names"=w562, "Units"=enum16{"Q l/min", "M_dot Kg/min"}."M_dot Kg/min", "Present scan array"=w561) -> ("Trace"=w558:dbl, "Carrier"=w559:dbl, "Scan comments"=w560:string)
          n189 = Add(x=w559, y=w558) -> (x+y=w556:dbl)
        }
        frame "GMU:Source:Meas Density" {
          n190 = Build Array("GMU:Source:Meas M_dot", "GMU:Source:Meas Q") -> (w568:string[])
          n191 = call "Read_Earlier_Channels.vi"("Present scan array"=w566, "Ch names"=w567, "Desired Channels"=w568) -> ("Scan comments"=w565:string, "Index 0"=w564:dbl, "Index 1"=w563:dbl)  [unwired: 3 out]
          n192 = Not Equal To 0?(x=w564) -> (x != 0?=w572:bool)
          n193 = case shown="False" w572 {
            tunnel: w564 -> [_ w576]
            tunnel: w563 -> [_ w575]
            tunnel: [0.0 w574] -> w571
            frame False {
            }
            frame True {
              n194 = Divide(x=w576, y=w575) -> (x/y=w577:dbl)
              n195 = Multiply(x=w577, y=1000.0) -> (x*y=w574:dbl)
            }
          }
        }
        frame "GMU:Source:Meas Den Ratio" {
          n196 = call "Read_value_of_earlier_Ch.vi"("Desired Ch to Read"="GMU:Source:Meas Density", "Ch names"=w585, "Present scan array"=w586) -> ("Value"=w581:dbl, "Scan comment"=w580:string)  [unwired: 1 in]
          n197 = Equal?(x=w581, y=w579) -> (x = y?=w583:bool)
          n198 = case shown="False" w583 {
            tunnel: w581 -> [w588 _]
            tunnel: [w587 w593] -> w582
            tunnel: w579 -> [_ w593]
            frame False {
              n199 = global read "Gas_management_global.vi" "Release temp (deg C)"() -> (w591:dbl)
              n200 = global read "Gas_management_global.vi" "Atmos Pres (mbars)"() -> (w590:dbl)
              n201 = call "Gas_Density.vi"("Pressure (mbars)"=w590, "Temperature (deg C)"=w591, "Gas Name"="Air") -> ("Density Kg/m3"=w589:dbl)
              n202 = Divide(x=w588, y=w589) -> (x/y=w587:dbl)
            }
            frame True {
            }
          }
        }
        frame "GMU:Source:Meas Strength" {
          n203 = call "Calculate_Release_Flowrates.vi"("Ch names"=w609, "Units"=enum16{"Q l/min", "M_dot Kg/min"}."Q l/min", "Present scan array"=w608) -> ("Trace"=w601:dbl, "Carrier"=w602:dbl, "Scan comments"=w607:string)
          n204 = Equal To 0?(x=w602) -> (x = 0?=w604:bool)
          n205 = Equal To 0?(x=w601) -> (x = 0?=w605:bool)
          n206 = And(x=w604, y=w605) -> (x .and. y?=w603:bool)
          n207 = case shown="False" w603 {
            tunnel: w602 -> [w620 _]
            tunnel: w601 -> [w619 _]
            tunnel: [w618 0.0] -> w597
            frame False {
              n208 = Add(x=w620, y=w619) -> (x+y=w623:dbl)
              n209 = Divide(x=w619, y=w623) -> (x/y=w622:dbl)
              n210 = Multiply(x=w622, y=100.0) -> (x*y=w618:dbl)
            }
            frame True {
            }
          }
          n211 = while {
            tunnel: [w611] -> w594
            tunnel: [w612] -> w596
            tunnel: w597 -> [w617]
            shift-left: _ -> [w611]
            shift-left: _ -> [w616]
            shift-right: [w617] -> _
            stop <- FALSE continue-if-true
            w615 = 6.0 ("y")
            n212 = Less?(x=w616, y=w615) -> (x < y?=w614:bool)
            n213 = Less?(x=w611, y=w615) -> (x < y?=w613:bool)
            n214 = Or(x=w614, y=w613) -> (x .or. y?=w612:bool)
          }
          n215 = Greater?(x=w597, y=7.0) -> (0:w595:bool)
          n216 = And(x=w596, y=w595) -> (x .and. y?=w599:bool)
          n217 = Select(t=w594, s=w599, f=w597) -> (s? t:f=w598:dbl)
        }
        frame "EnFlo_Tunnel:Temp:Inlet_Av" {
          w632 = 0.0 ("Value")
          w626 = "EnFlo_Tunnel:Temp:Inlet"
          n218 = String Length(string=w626) -> (length=w627:i32)
          n219 = for {
            tunnel: w634 -> [w640] mode=indexing
            tunnel: w633 -> [w639] mode=indexing
            shift-right: [w647] -> w631
            shift-left: w632 -> [w646]
            shift-right: [w644] -> w630
            shift-left: w632 -> [w645]
            tunnel: w627 -> [w643]
            tunnel: w626 -> [w641]
            tunnel: "EnFlo_Tunnel:Temp:Inlet_Av" -> [w638]
            n220 = String Subset(string=w639, length (rest)=w643) -> (substring=w642:string)  [unwired: 1 out]
            n221 = Equal?(x=w642, y=w641) -> (x = y?=w636:bool)
            n222 = Not Equal?(x=w639, y=w638) -> (x != y?=w637:bool)
            n223 = And(x=w636, y=w637) -> (x .and. y?=w635:bool)
            n224 = case shown="True" w635 {
              tunnel: [w649 w653] -> w647
              tunnel: w646 -> [w649 w654]
              tunnel: w640 -> [_ w652]
              tunnel: w645 -> [w648 w651]
              tunnel: [w648 w650] -> w644
              frame False {
              }
              frame True {
                n225 = Add(x=w652, y=w654) -> (x+y=w653:dbl)
                n226 = Increment(x=w651) -> (x+1=w650:dbl)
              }
            }
          }
          n227 = Divide(x=w631, y=w630) -> (x/y=w629:dbl)
        }
        frame "EnFlo Lab:labstrat1:Av Temp" {
          w659 = 0.0 ("Value")
          n228 = for {
            tunnel: w663 -> [w675]
            tunnel: w662 -> [w674]
            shift-right: [w671] -> w660
            shift-left: "" -> [w672]
            shift-right: [w669] -> w658
            shift-left: w659 -> [w668]
            shift-right: [w665] -> w657
            shift-left: w659 -> [w666]
            tunnel: string[] ["EnFlo Lab:labstrat1:Z=4.5m", "EnFlo Lab:labstrat1:Z=3.5m", "EnFlo Lab:labstrat1:Z=2.5m", "EnFlo Lab:labstrat1:Z=1.5m", "EnFlo Lab:labstrat1:Z=0.5m"] -> [w664] mode=indexing
            n229 = call "Read_value_of_earlier_Ch.vi"("Desired Ch to Read"=w664, "Ch names"=w674, "Present scan array"=w675) -> ("Value"=w667:dbl, "Scan comment"=w673:string)  [unwired: 1 in]
            n230 = Concatenate Strings(w672, w673) -> (w671:string)
            n231 = Not A Number/Path/Refnum?(number/path/refnum=w667) -> (NaN/Path/Refnum?=w670:bool)
            n232 = case shown="True" w670 {
              tunnel: [w679 w682] -> w669
              tunnel: w668 -> [w680 w682]
              tunnel: w667 -> [w678 _]
              tunnel: w666 -> [w677 w681]
              tunnel: [w676 w681] -> w665
              frame False {
                n233 = Add(x=w678, y=w680) -> (x+y=w679:dbl)
                n234 = Increment(x=w677) -> (x+1=w676:dbl)
              }
              frame True {
              }
            }
          }
          n235 = Divide(x=w658, y=w657) -> (x/y=w656:dbl)
        }
        frame "EnFlo Lab:labstrat1:Delta T" {
          n236 = Build Array("EnFlo Lab:labstrat1:Z=4.5m", "EnFlo Lab:labstrat1:Z=0.5m") -> (w690:string[])
          n237 = call "Read_Earlier_Channels.vi"("Present scan array"=w686, "Ch names"=w687, "Desired Channels"=w690) -> ("Scan comments"=w685:string, "Index 0"=w684:dbl, "Index 1"=w683:dbl)  [unwired: 3 out]
          n238 = Subtract(x=w684, y=w683) -> (x-y=w691:dbl)
        }
        frame "Laser:Cooling_Water:Delta_T" {
          n239 = Build Array("LDA Laser:Cooling water:Return Temp", "LDA Laser:Cooling water:Supply Temp") -> (w699:string[])
          n240 = call "Read_Earlier_Channels.vi"("Present scan array"=w695, "Ch names"=w696, "Desired Channels"=w699) -> ("Scan comments"=w694:string, "Index 0"=w693:dbl, "Index 1"=w692:dbl)  [unwired: 3 out]
          n241 = Subtract(x=w693, y=w692) -> (x-y=w700:dbl)
        }
        frame "EnFlo_Tunnel:Chilled Water:Valve Dem Pos" {
          n242 = Get Date/Time In Seconds() -> (seconds since 1Jan1904=w702:timestamp)
          n243 = Concatenate Strings(w703, " last updated") -> (w711:string)
          n244 = To Double Precision Float(number=w702) -> (double precision float=w701:dbl)
          n245 = Unbundle By Name(w709) -> ("A"=w708:dbl)
          n246 = call "Remember_value.vi"("Mode"=Remember_value_mode."Read only", "Ch name"=w711) -> ("Output Value"=w710:dbl)  [unwired: 1 in]
          n247 = Subtract(x=w701, y=w710) -> (x-y=w707:dbl)
          n248 = Greater?(x=w707, y=w708) -> (0:w706:bool)
          n249 = Not A Number/Path/Refnum?(number/path/refnum=w707) -> (NaN/Path/Refnum?=w705:bool)
          n250 = Or(x=w705, y=w706) -> (x .or. y?=w704:bool)
          n251 = case shown="True" w704 {
            tunnel: w718 -> [w719 w738]
            tunnel: [w719 w737] -> w717
            tunnel: w716 -> [_ w729]
            tunnel: w715 -> [_ w730]
            tunnel: ["" w735] -> w714
            tunnel: w711 -> [_ w725]
            tunnel: w701 -> [_ w721]
            frame False {
            }
            frame True {
              n252 = call "Read_value_of_earlier_Ch.vi"("Desired Ch to Read"="EnFlo_Tunnel:Chiller_Pump:Enable", "Ch names"=w730, "Present scan array"=w729) -> ("Value"=w728:dbl)  [unwired: 1 in, 1 out]
              n253 = Build Array("EnFlo_Tunnel:Chilled Water:Dem Temp", "EnFlo_Tunnel:Chilled Water:Supply", "EnFlo_Tunnel:Chiller_Pump:Running") -> (w736:string[])
              n254 = call "Read_Earlier_Channels.vi"("Present scan array"=w729, "Ch names"=w730, "Desired Channels"=w736) -> ("Scan comments"=w735:string, "Index 0"=w734:dbl, "Index 1"=w733:dbl, "Index 2"=w723:dbl)  [unwired: 2 out]
              n255 = Greater?(x=w728, y=0.5) -> (0:w726:bool)
              n256 = Greater?(x=w723, y=0.5) -> (0:w722:bool)
              n257 = case shown="False" w722 {
                tunnel: w738 -> [_ w766]
                tunnel: [w753 w760] -> w737
                tunnel: w734 -> [_ w762]
                tunnel: w733 -> [_ w761]
                tunnel: w721 -> [_ w759]
                tunnel: w726 -> [w744 _]
                tunnel: w725 -> [_ w758]
                frame False {
                  n258 = Seconds To Date/Time() -> (date time rec=w741:T13)  [unwired: 2 out]
                  n259 = Unbundle By Name(w741) -> ("day of week"=w748:i32, "hour"=w750:i32)
                  n260 = Less?(x=w750, y=3) -> (x < y?=w745:bool)
                  n261 = Equal?(x=7, y=w748) -> (x = y?=w746:bool)
                  n262 = And(x=w746, y=w745) -> (x .and. y?=w743:bool)
                  n263 = case shown="True" w744 {
                    tunnel: w743 -> [w754 w756]
                    tunnel: [w754 w755] -> w742
                    frame False {
                    }
                    frame True {
                      n264 = Not(x=w756) -> (.not. x?=w755:bool)
                    }
                  }
                  n265 = Select(t=0.0, s=w742, f=100.0) -> (s? t:f=w753:dbl)
                }
                frame True {
                  w764 = 100.0  # Max
                  w765 = 0.0  # Min
                  n266 = call "PID.vi"("Present Value"=w761, "Previous Control Sum"=w766, "Setpoint"=w762) -> ("Dem Output"=w763:dbl)
                  n267 = In Range and Coerce(upper limit=w764, x=w763, lower limit=w765) -> (coerced(x)=w760:dbl)  [unwired: 1 out]
                  n268 = call "Remember_value.vi"("Mode"=Remember_value_mode."Read and Write", "Input Value"=w759, "Ch name"=w758) -> ()  [unwired: 1 out]
                }
              }
            }
          }
        }
        frame "EnFlo_Tunnel:Hydrosonic:Integral" {
          n269 = Build Array("EnFlo_Tunnel:Usonic Fixed:Velocity", "Hydrosonic:Transducer:Setting") -> (w776:string[])
          n270 = call "Read_Earlier_Channels.vi"("Present scan array"=w777, "Ch names"=w775, "Desired Channels"=w776) -> ("Scan comments"=w769:string, "Index 0"=w774:dbl, "Index 1"=w768:dbl)  [unwired: 3 out]
          n271 = Greater?(x=w774, y=0.5) -> (0:w772:bool)
          n272 = case shown="True" w772 {
            tunnel: w771 -> [w780 w788]
            tunnel: [w780 w787] -> w770
            tunnel: w768 -> [_ w786]
            tunnel: w767 -> [_ w785]
            frame False {
            }
            frame True {
              w783 = 8640000.0  # Seconds per day x 100
              n273 = Multiply(x=w786, y=w785) -> (x*y=w784:dbl)
              n274 = Divide(x=w784, y=w783) -> (x/y=w782:dbl)
              n275 = Not A Number/Path/Refnum?(number/path/refnum=w782) -> (NaN/Path/Refnum?=w781:bool)
              n276 = case shown="False" w781 {
                tunnel: w788 -> [w791 w792]
                tunnel: [w790 w792] -> w787
                tunnel: w782 -> [w789 _]
                frame False {
                  n277 = Add(x=w789, y=w791) -> (x+y=w790:dbl)
                }
                frame True {
                }
              }
            }
          }
        }
        frame "EnFlo_Tunnel:Days Run at:2.5m/s" {
          n278 = Build Array("EnFlo_Tunnel:Usonic Fixed:Velocity") -> (w801:string[])
          n279 = call "Read_Earlier_Channels.vi"("Present scan array"=w802, "Ch names"=w800, "Desired Channels"=w801) -> ("Scan comments"=w795:string, "Index 0"=w793:dbl)  [unwired: 4 out]
          n280 = Greater?(x=w793, y=0.5) -> (0:w798:bool)
          n281 = case shown="True" w798 {
            tunnel: w797 -> [w804 w812]
            tunnel: [w804 w811] -> w796
            tunnel: w793 -> [_ w810]
            tunnel: w794 -> [_ w809]
            frame False {
            }
            frame True {
              w807 = 216000.0  # Seconds per day x 2.5
              n282 = Multiply(x=w810, y=w809) -> (x*y=w808:dbl)
              n283 = Divide(x=w808, y=w807) -> (x/y=w806:dbl)
              n284 = Not A Number/Path/Refnum?(number/path/refnum=w806) -> (NaN/Path/Refnum?=w805:bool)
              n285 = case shown="True" w805 {
                tunnel: w812 -> [w815 w816]
                tunnel: [w814 w816] -> w811
                tunnel: w806 -> [w813 _]
                frame False {
                  n286 = Add(x=w813, y=w815) -> (x+y=w814:dbl)
                }
                frame True {
                }
              }
            }
          }
        }
        frame "Complete:Scan:Period" {
          n287 = while {
            tunnel: [w826] -> w819
            tunnel: [w833] -> w821
            shift-left: _ -> [w833]
            shift-right: [w834] -> w822
            tunnel: w818 -> [w830]
            tunnel: [w825] -> w817
            stop <- FALSE continue-if-true
            w825 = 10.0 ("Averaging time (mins)")
            n288 = Build Array(w830) -> (w829:string[])
            n289 = call "Get_Channel_averages.vi"("Desired Ch Names"=w829, "Averaging time (mins)"=w825) -> ("number"=w828:dbl[])  [unwired: 1 in, 2 out]
            n290 = Index Array(array=w828, index=0) -> (element=w826:dbl)
            n291 = Greater?(x=w826, y=20.0) -> (0:w834:bool)
          }
          n292 = Compound Arithmetic op=AND(w822, invert w821) -> (w820:bool)
          n293 = case shown="True" w820 {
            tunnel: w819 -> [_ w840]
            tunnel: w817 -> [_ w835]
            frame False {
            }
            frame True {
              n294 = Format Into String(format string="Warning! The average scan period on the ADAM Scan table is %.1f seconds over the last %d minutes." ("Format String"), w840, w835) -> (resulting string=w838:string)  [unwired: 2 in, 1 out]
              n295 = call "Server_Emails.vi"("Message"=w838, "Contact All clients?"=TRUE, "Subject"="Scan Period") -> ()  [unwired: 2 in, 3 out]
            }
          }
        }
        frame "GMU:Source:Est Time" {
          # "NaN's"
          # "Est?"
          # "Inband?"
          n296 = stacked-sequence {
            seq-local: [w847 _ _ _] -> [_ _ w894 _]
            seq-local: [_ w859 _ _] -> [_ _ w891 _]
            seq-local: [_ w860 _ _] -> [_ _ w889 _]
            seq-local: [_ _ w896 _] -> [_ _ _ w912]
            seq-local: [w851 _ _ _] -> [_ _ w893 _]
            seq-local: [_ w858 _ _] -> [_ _ _ w908]
            tunnel: w846 -> [w853 w861 w899 _]
            tunnel: w845 -> [w852 w862 w900 _]
            tunnel: [_ _ w892 _] -> w844
            tunnel: [_ _ _ w911] -> w843
            tunnel: w842 -> [_ _ _ w910]
            tunnel: w841 -> [_ _ _ w909]
            frame #0 {
              n297 = Build Array("GMU:Source:Density Ratio", "GMU:Source:Dem Strength", "GMU:Source:Dem Q") -> (w854:string[])
              n298 = call "Read_Earlier_Channels.vi"("Present scan array"=w852, "Ch names"=w853, "Desired Channels"=w854) -> ("Scan comments"=w851:string, "Index 0"=w850:dbl, "Index 1"=w849:dbl, "Index 2"=w848:dbl)  [unwired: 2 out]
              n299 = Build Array(w850, w849, w848) -> (w847:dbl[])
            }
            frame #1 {
              n300 = for {
                N: 2 -> [_]
                tunnel: w862 -> [w872]
                tunnel: w861 -> [w873]
                tunnel: [w871] -> w859 mode=indexing
                tunnel: [w878] -> w860 mode=indexing
                tunnel: [w877] -> w858 mode=indexing
                i -> [w883]
                w882 = 23.0  # %
                n301 = case shown="1" w883 {
                  tunnel: ["GMU:Source:Meas Q" "GMU:Source:Meas Strength"] -> w876
                  tunnel: ["GMU:Source:Dem Q" "GMU:Source:Dem Strength"] -> w875
                  frame 0, Default {
                  }
                  frame 1 {
                  }
                }
                n302 = Build Array(w875, w876) -> (w874:string[])
                n303 = call "Read_Earlier_Channels.vi"("Present scan array"=w872, "Ch names"=w873, "Desired Channels"=w874) -> ("Scan comments"=w871:string, "Index 0"=w869:dbl, "Index 1"=w870:dbl)  [unwired: 3 out]
                n304 = Not A Number/Path/Refnum?(number/path/refnum=w870) -> (NaN/Path/Refnum?=w877:bool)
                n305 = Subtract(x=w870, y=w869) -> (x-y=w868:dbl)
                n306 = Greater Than 0?(x=w869) -> (x > 0?=w879:bool)
                n307 = Less?(x=w868, y=0.05) -> (x < y?=w865:bool)
                n308 = call "In_Range_check.vi"("%"=w882, "Mode"=In_Range."%", "Value"=w870, "Setpoint"=w869) -> ("In Range"=w866:bool)  [unwired: 1 in, 2 out]
                n309 = Or(x=w866, y=w865) -> (x .or. y?=w864:bool)
                n310 = And(x=w864, y=w879) -> (x .and. y?=w880:bool)
                n311 = Compound Arithmetic op=OR(w880, invert w879, w877) -> (w878:bool)
              }
            }
            frame #2 {
              n312 = while {
                tunnel: [w907] -> w895
                tunnel: w894 -> [w906]
                shift-left: _ -> [w907]
                shift-right: [w906] -> _
                stop <- FALSE continue-if-true
              }
              n313 = Equal?(x=w894, y=w895) -> (x = y?=w901:bool)
              n314 = call "Read_value_of_earlier_Ch.vi"("Desired Ch to Read"="GMU:Source:Dem Q", "Ch names"=w899, "Present scan array"=w900) -> ("Value"=w897:dbl)  [unwired: 1 in, 1 out]
              n315 = Greater Than 0?(x=w897) -> (x > 0?=w904:bool)
              n316 = And Array Elements(Boolean array=w889) -> (logical AND=w888:bool)
              n317 = Select(t=w888, s=w904, f=TRUE) -> (s? t:f=w902:bool)
              n318 = Compound Arithmetic op=AND(w901, w902) -> (w896:bool)
              n319 = Concatenate Strings(w891) -> (w890:string)
              n320 = Concatenate Strings(w890, w893) -> (w892:string)
            }
            frame #3 {
              n321 = case shown="True" w912 {
                tunnel: [0.0 w914] -> w911
                tunnel: w910 -> [_ w919]
                tunnel: w909 -> [_ w915]
                tunnel: w908 -> [_ w918]
                frame False {
                }
                frame True {
                  n322 = Or Array Elements(Boolean array=w918) -> (logical OR=w917:bool)
                  n323 = Add(x=w919, y=w915) -> (x+y=w916:dbl)
                  n324 = Select(t=w915, s=w917, f=w916) -> (s? t:f=w914:dbl)
                }
              }
            }
          }
        }
      }
    }
    frame "Hold Value" {
    }
    frame "Read A" {
      n325 = Unbundle By Name(w923) -> ("A"=w922:dbl)
    }
    frame "Read Ch" {
      n326 = Unbundle By Name(w928) -> ("String"=w925:string)
      n327 = call "Read_value_of_earlier_Ch.vi"("Desired Ch to Read"=w925, "Ch names"=w929, "Present scan array"=w930) -> ("Value"=w926:dbl, "Scan comment"=w927:string)  [unwired: 1 in]
    }
    frame "Coded" {
    }
    frame "Client Info" {
      n328 = global read "ADAM_Global.vi" "Client State Array"() -> (w945:T14[])
      n329 = call "Split_Ch_name.vi"("Ch name"=w939) -> ("Top level"=w937:string, "Low level"=w935:string)  [unwired: 1 out]
      n330 = Equal?(x="Status" ("Substring"), y=w937) -> (x = y?=w936:bool)
      n331 = Select(t=w935, s=w936, f="") -> (s? t:f=w933:string)
      n332 = for {
        tunnel: w945 -> [w954] mode=indexing
        tunnel: [w953] -> w946 mode=indexing
        n333 = Unbundle By Name(w954) -> ("Client Name"=w953:string)
      }
      n334 = Search 1D Array(1D array=w946, element=w933) -> (index of element=w941:i32)  [unwired: 1 out]
      n335 = Less Than 0?(x=w941) -> (x < 0?=w940:bool)
      n336 = Index Array(array=w945, index=w941) -> (element=w944:T14)
      n337 = case shown="False" w940 {
        tunnel: w944 -> [w949 _]
        tunnel: w933 -> [w948 w951]
        tunnel: [w947 w950] -> w943
        frame False {
          n338 = call "Get_Client_Status_string.vi"("Client State Cluster"=w949, "Client Name"=w948) -> ("Code Value"=w947:dbl)  [unwired: 1 in]
        }
        frame True {
          w950 = 7.0 ("Code Value")
          n339 = call "Remember_value.vi"("Mode"=Remember_value_mode."Read and Write", "Input Value"=w950, "Ch name"=w951) -> ()  [unwired: 1 out]
        }
      }
    }
    frame "Web Client" {
      w964 = 7200.0  # 2 Hours in Seconds
      n340 = Concatenate Strings(w973, ":Last read" ("Substring")) -> (w971:string)
      n341 = call "Remember_value.vi"("Mode"=Remember_value_mode."Read only", "Ch name"=w971) -> ("Output Value"=w970:dbl)  [unwired: 1 in]
      n342 = Not A Number/Path/Refnum?(number/path/refnum=w970) -> (NaN/Path/Refnum?=w968:bool)
      n343 = Get Date/Time In Seconds() -> (seconds since 1Jan1904=w963:timestamp)
      n344 = To Double Precision Float(number=w963) -> (double precision float=w961:dbl)
      n345 = Subtract(x=w961, y=w970) -> (x-y=w976:dbl)
      n346 = Greater?(x=w976, y=1800.0) -> (0:w969:bool)
      n347 = Or(x=w969, y=w968) -> (x .or. y?=w955:bool)
      n348 = case shown="True" w955 {
        frame False {
        }
        frame True {
          n349 = global read "Constants_global.vi" "EnFlo SW Folder"() -> (w979:path)
          n350 = Build Path(base path=w979, name or relative path=path "ADAM Server/Sub VI's/Web_Client.vi") -> (appended path=w978:path)
          n351 = Open VI Reference(vi path=w978) -> (vi reference=w983:refnum<vi>, error out=w984:errorcluster)  [unwired: 1 in, 4 out]
          n352 = property class="VI"(reference=w983, error in=w984) -> (reference out=w986:refnum<vi>, error out=w987:errorcluster, "Front Panel Window:Open"=w985:bool)
          n353 = case shown="False" w985 {
            tunnel: w986 -> [w993 w996]
            tunnel: w987 -> [w992 w995]
            tunnel: [w991 w996] -> w988
            tunnel: [w990 w995] -> w989
            frame False {
              n354 = property class="VI"(reference=w993, error in=w992, "Front Panel Window:Open"=TRUE) -> (reference out=w991:refnum<vi>, error out=w990:errorcluster)
            }
            frame True {
            }
          }
          n355 = invoke class="VI" method="Run VI"(reference=w988, error in=w989, "Wait until done"=FALSE, "Auto Dispose Ref"=TRUE) -> ()  [unwired: 1 in, 5 out]
        }
      }
      n356 = Concatenate Strings(w973, ":value time" ("Substring")) -> (w957:string)
      n357 = call "Remember_value.vi"("Mode"=Remember_value_mode."Read only", "Ch name"=w973) -> ("Output Value"=w977:dbl)  [unwired: 1 in]
      n358 = call "Remember_value.vi"("Mode"=Remember_value_mode."Read only", "Ch name"=w957) -> ("Output Value"=w962:dbl)  [unwired: 1 in]
      n359 = Subtract(x=w961, y=w962) -> (x-y=w960:dbl)
      n360 = Greater?(x=w960, y=w964) -> (0:w967:bool)
      n361 = case shown="True" w967 {
        tunnel: w960 -> [_ w1002]
        tunnel: 3600.0 ("y") -> [_ w1001]
        tunnel: ["" w999] -> w966
        frame False {
        }
        frame True {
          n362 = Divide(x=w1002, y=w1001) -> (x/y=w998:dbl)
          n363 = Format Into String(format string="Value is %d hours old." ("Format String"), w998) -> (resulting string=w999:string)  [unwired: 2 in, 1 out]
        }
      }
    }
    frame "X10" {
      (unwired) 1 items=["-----", "A", "B", "C", "D", "E", "F", "G", "H", "I", "J", "K", "L", "M", "N", "O", "P"] ("House Code")
      n364 = Greater Than 0?(x=w1007) -> (x > 0?=w1006:bool)
      n365 = Unbundle By Name(w1012) -> ("Port Name"=w1009:string, "Main"=w1010:i32, "Ch."=w1011:i32)
      n366 = call "X10control.vi"("Port Name"=w1009, "Power Request (ON)"=w1006, "House Code"=w1010, "Unit No."=w1011) -> ()  [unwired: 6 out]
      n367 = Select(t=1.0, s=w1006, f=0.0) -> (s? t:f=w1003:dbl)
    }
    frame "Test" {
      n368 = case shown="True" "Case Constant\n(See Context Help) 2" {
        tunnel: [w1020 w1027] -> w1017
        tunnel: ["Crazy time based random number!" w1028] -> w1016
        tunnel: w1015 -> [_ w1030]
        tunnel: w1014 -> [_ w1029]
        frame False {
          w1023 = 0.0005  # y
          n369 = Get Date/Time In Seconds() -> (seconds since 1Jan1904=w1018:timestamp)
          n370 = To Double Precision Float(number=w1018) -> (double precision float=w1025:dbl)
          n371 = Subtract(x=w1025, y=2969882881.0) -> (x-y=w1024:dbl)
          n372 = Multiply(x=w1024, y=w1023) -> (x*y=w1021:dbl)
          n373 = Random Number (0-1)() -> (number: 0 to 1=w1022:dbl)
          n374 = Add(x=w1022, y=w1021) -> (x+y=w1020:dbl)
        }
        frame True {
          n375 = call "LPA400_get_rdg.vi"("Channel Name"=w1029, "Address"=w1030) -> ("Output"=w1027:dbl, "Status note"=w1028:string)  [unwired: 4 out]
        }
      }
    }
  }
  "Output" <- w8
  "Scan comment" <- w5
